vi "Init Sync Stuff.vi"(8 "error in (no error)":errorcluster, 10 "IO-4 Bricklet in":refnum<class "IO-4 Bricklet.lvclass">) -> (0 "error out":errorcluster, 2 "IO-4 Bricklet out":refnum<class "IO-4 Bricklet.lvclass">)   [LabVIEW 2011, in "Tinkerforge.lvlib" / "IO-4 Bricklet.lvclass"]
doc: "This VI is the child implementation of \"Init Sync Stuff.vi\" and initializes all synchronization objects of this child object."
uses:
  IO-4 Bricklet.lvclass
  Type Definitions/Interrupt.ctl
  IO-4 Bricklet.lvclass/IO-4 Bricklet.ctl
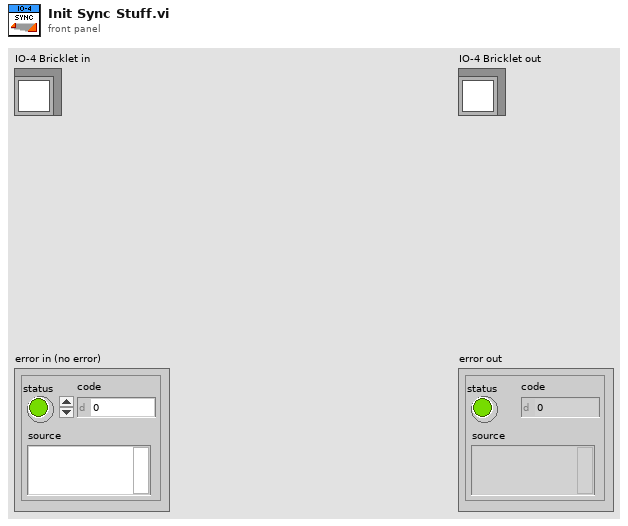
[diagram p1: front panel]
types:
  T1 = typedef "Tinkerforge.lvlib/IO-4 Bricklet.lvclass/Interrupt.ctl" = cluster{"Interrupt Mask":u8, "Value Mask":u8}
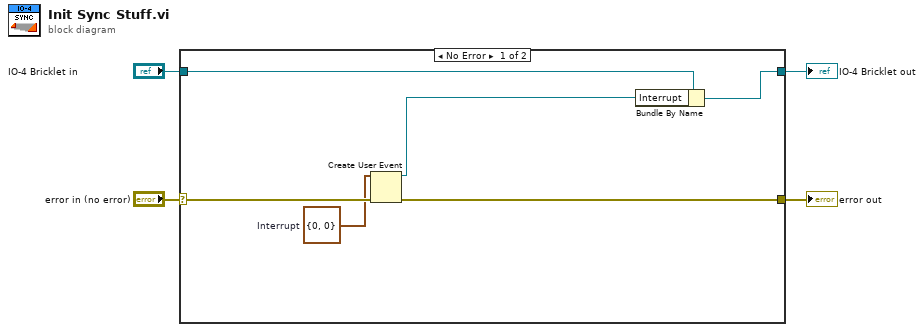
[diagram p0: block diagram]
diagram:
  n1 = case shown="No Error" "error in (no error)" {
    selector: "error in (no error)" -> [w10 w11]
    tunnel: "IO-4 Bricklet in" -> [w6 w12]
    tunnel: [w7 w11] -> w2
    tunnel: [w9 w12] -> w1
    frame No Error {
      w5 = T1 {"Interrupt Mask"=0, "Value Mask"=0}  # Interrupt
      n2 = Create User Event(user event datatype=w5, error in=w10) -> (user event=w8:refnum<user-event>, error out=w7:errorcluster)
      n3 = Bundle By Name(cluster=w6, "Interrupt"=w8) -> (w9:refnum<class "IO-4 Bricklet.lvclass">)
    }
    frame Error {
    }
  }
  "error out" <- w2
  "IO-4 Bricklet out" <- w1
